vi "Write shared variable IR_data.vi"(8 "error in (no error)":errorcluster, 10 "shared variable IR_data":refnum<k21>, 11 "VIS-NIR_STRESING_NEW in":refnum<class "VIS-NIR_STRESING_NEW.lvclass">) -> (0 "error out":errorcluster, 3 "VIS-NIR_STRESING_NEW out":refnum<class "VIS-NIR_STRESING_NEW.lvclass">)   [LabVIEW 2020, in "VIS-NIR_STRESING_NEW.lvclass"]
uses:
  VIS-NIR_STRESING_NEW/VIS-NIR_STRESING_NEW.lvclass
  VIS-NIR_STRESING_NEW/VIS-NIR_STRESING_NEW.lvclass/VIS-NIR_STRESING_NEW.ctl
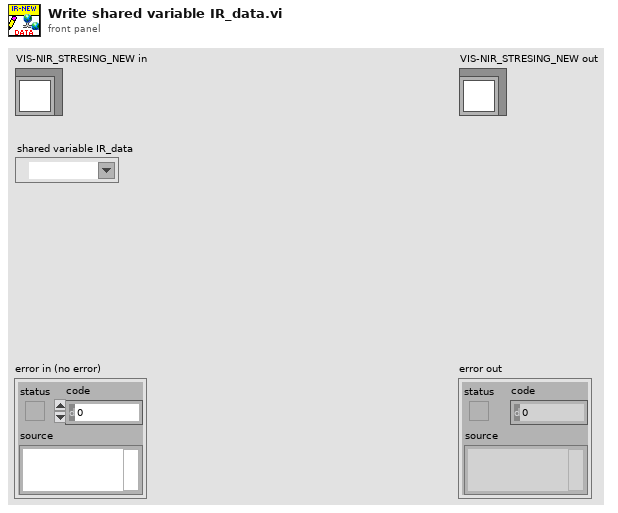
[diagram p1: front panel]
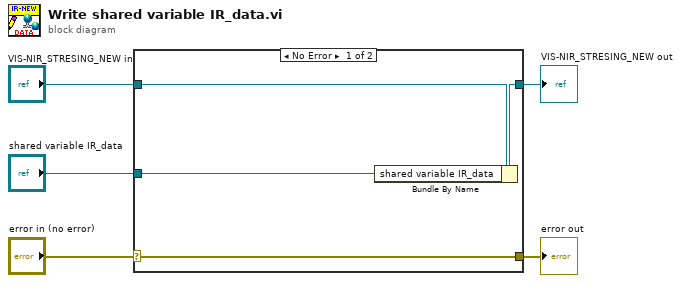
[diagram p0: block diagram]
diagram:
  n1 = case shown="No Error" "error in (no error)" {
    selector: "error in (no error)" -> [w9 w10]
    tunnel: [w9 w10] -> w4
    tunnel: [w7 w11] -> w2
    tunnel: "VIS-NIR_STRESING_NEW in" -> [w8 w11]
    tunnel: "shared variable IR_data" -> [w6 _]
    frame No Error {
      n2 = Bundle By Name(cluster=w8, "shared variable IR_data"=w6) -> (w7:refnum<class "VIS-NIR_STRESING_NEW.lvclass">)
    }
    frame Error {
    }
  }
  "error out" <- w4
  "VIS-NIR_STRESING_NEW out" <- w2
